vi "Get Absolute XY.vi"(8 "error in (no error)":errorcluster, 10 "Component":T1, 11 "Gantry In":refnum<k24>) -> (0 "error out":errorcluster, 2 "Abs XY":dbl[](array[numeric]), 3 "Gantry Out":refnum<k24>)   [LabVIEW 2021, in "Component Tray.lvclass"]
uses:
  Component Tray.lvclass
  C:/Program Files (x86)/Aerotech/A3200/LabVIEW/2010/Bin/Aerotech.A3200.dll
  Program Files (x86)/Aerotech/A3200/LabVIEW/2010/Bin/Aerotech.A3200.dll
  Find Component.ctl
  Controller/Camera/Machine Vision.ctl
  Component Tray.lvclass/Component Tray.ctl
  Controller/Motion/A3200/A3200.lvclass
  Controller/Camera/Camera.lvclass
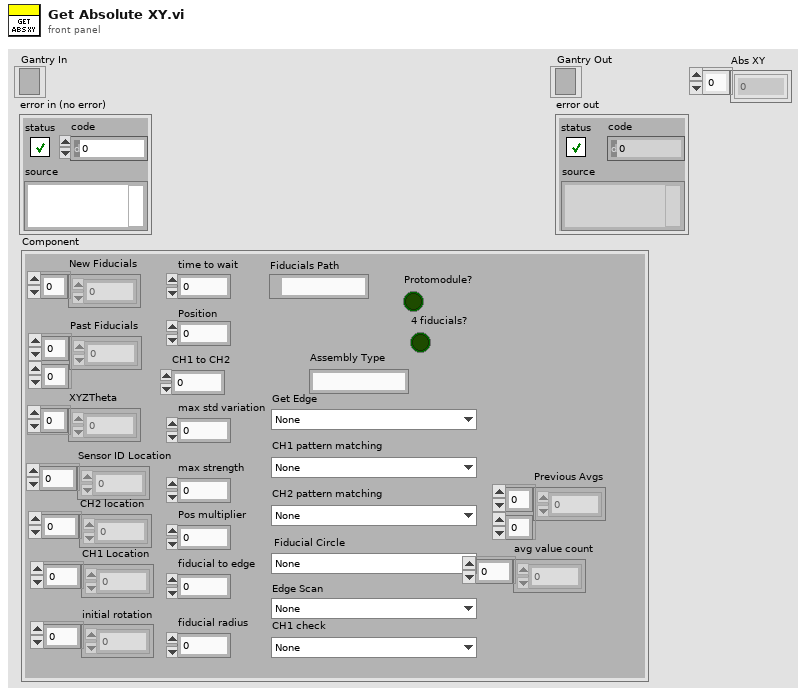
[diagram p1: front panel]
types:
  T1 = typedef "Component Tray.lvclass/Find Component.ctl" = cluster{"New Fiducials":dbl[], "Past Fiducials":dbl[][], "XYZTheta":dbl[], "Fiducials Path":path, "Position":i32, "CH1 Location":dbl[], "Sensor ID Location":dbl[], "initial rotation":dbl[], "CH2 location":dbl[], "max std variation":dbl, "max strength":dbl, "CH2 pattern matching":T2, "Fiducial Circle":T2, "Get Edge":T2, "Pos multiplier":dbl, "time to wait":u32, "fiducial to edge":dbl, "Protomodule?":bool, "Assembly Type":string, "CH1 to CH2":dbl, "Tray Number":string, "fiducial radius":dbl, "4 fiducials?":bool, "CH1 check":T2, "Edge Scan":T2, "CH1 pattern matching":T2, "Sensor Thickness":dbl, "Previous Avgs":dbl[][], "avg value count":dbl[]}
  T2 = typedef "Camera.lvclass/Machine Vision.ctl" = enum16{"None", "Assembly Tray Circle", "Assembly Tray Fiducial", "Partial Hexaboard", "sensor edge init", "HB edge init", "sensor edge pos1", "sensor edge pos2", "HB edge pos1", "HB edge pos2", "Sensor CH1-2", "HB CH1", "HB CH2", "V3 Sensor Circle", "Hexaboard Circle", "sensor CH1 check", "HB CH1 check ", "sensor ID"}
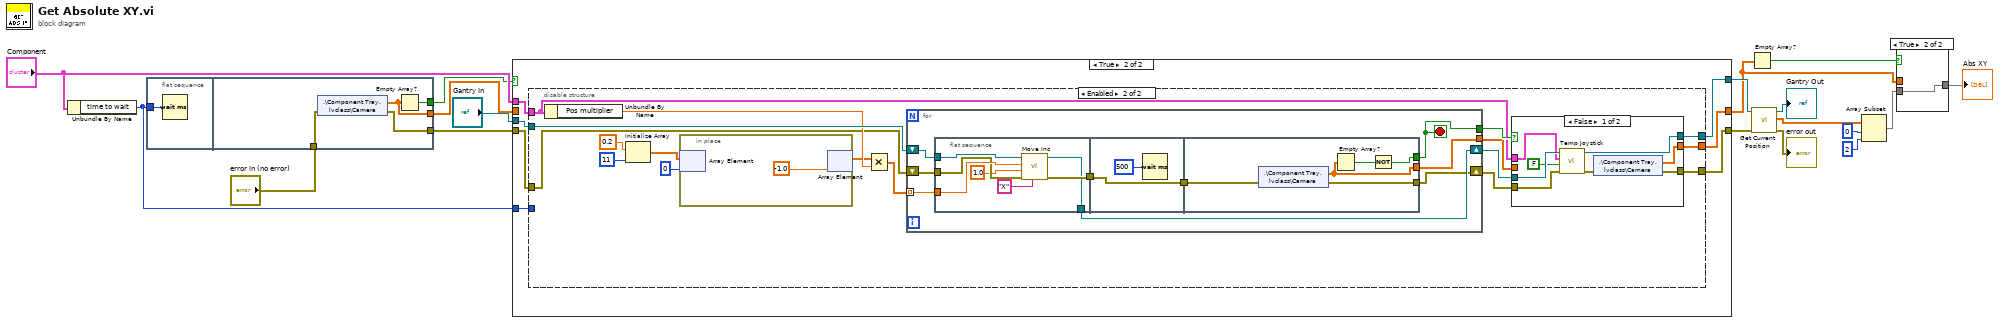
[diagram p0: block diagram]
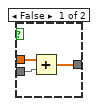
[diagram p2: hidden frame]
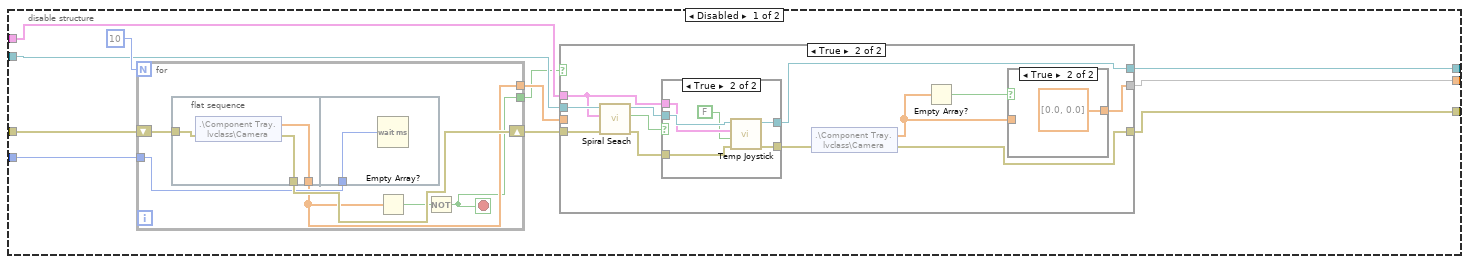
[diagram p4: hidden frame]
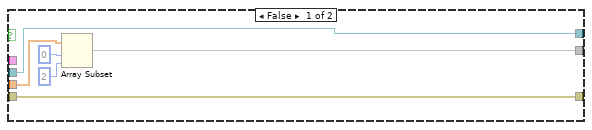
[diagram p5: hidden frame]
diagram:
  n1 = Unbundle By Name("Component") -> ("time to wait"=w11:u32)
  n2 = flat-sequence {
    tunnel: w11 -> [w19]
    tunnel: "error in (no error)" -> [w23]
    tunnel: [w22] -> w9
    tunnel: [w21] -> w8
    tunnel: [w20] -> w7
    frame #0 {
      n3 = Wait (ms)(milliseconds to wait=w19) -> ()  [unwired: 1 out]
    }
    frame #1 {
      n4 = shared-variable ".\\Component Tray.lvclass\\Camera"(error in=w23) -> (w22:dbl[], error out=w21:errorcluster)
      n5 = Empty Array?(array=w22) -> (empty?=w20:bool)
    }
  }
  n6 = case shown="True" w7 {
    tunnel: [w24 w32] -> w2
    tunnel: w8 -> [w26 w33]
    tunnel: [w26 w27] -> w6
    tunnel: w11 -> [_ w31]
    tunnel: "Gantry In" -> [w25 w30]
    tunnel: [w25 w29] -> w12
    tunnel: "Component" -> [_ w28]
    tunnel: w9 -> [w24 _]
    frame False {
    }
    frame True {
      n7 = disable-structure shown="Enabled" {
        disable-tunnel: w33 -> [w43 w96]
        disable-tunnel: [w41 w83] -> w32
        disable-tunnel: w31 -> [w40 _]
        disable-tunnel: w30 -> [w39 w99]
        disable-tunnel: [w38 w93] -> w29
        disable-tunnel: w28 -> [w37 w92]
        disable-tunnel: [w35 w90] -> w27
        frame Disabled {
          n8 = for {
            N: 10 -> [_]
            shift-right: [w49] -> w36
            shift-left: w43 -> [w50]
            tunnel: [w47] -> w42
            tunnel: w40 -> [w48]
            tunnel: [w45] -> w34
            stop <- w45 stop-if-true
            n9 = flat-sequence {
              tunnel: w50 -> [w53]
              tunnel: [w52] -> w49
              tunnel: [w51] -> w47
              tunnel: w48 -> [w54]
              frame #0 {
                n10 = shared-variable ".\\Component Tray.lvclass\\Camera"(error in=w53) -> (w51:dbl[], error out=w52:errorcluster)
              }
              frame #1 {
                n11 = Wait (ms)(milliseconds to wait=w54) -> ()  [unwired: 1 out]
              }
            }
            n12 = Empty Array?(array=w47) -> (empty?=w46:bool)
            n13 = Not(x=w46) -> (.not. x?=w45:bool)
          }
          n14 = case shown="True" w34 {
            tunnel: w42 -> [w58 _]
            tunnel: [w57 w61] -> w41
            tunnel: w39 -> [w56 w72]
            tunnel: [w56 w68] -> w38
            tunnel: w37 -> [_ w66]
            tunnel: w36 -> [w55 w71]
            tunnel: [w55 w64] -> w35
            frame False {
              n15 = Array Subset(array=w58, index=0, length=2) -> (w57:dbl[])
            }
            frame True {
              n16 = call "Spiral Seach.vi"("error in (no error)"=w71, "Component"=w66, "Gantry In"=w72) -> ("error out"=w67:errorcluster, "Error?"=w70:bool, "Gantry Out"=w69:refnum<k24>)  [unwired: 6 in]
              n17 = case shown="True" w70 {
                tunnel: w69 -> [w76 w82]
                tunnel: [w76 w81] -> w68
                tunnel: w67 -> [w75 w80]
                tunnel: [w75 w79] -> w65
                tunnel: w66 -> [_ w78]
                frame False {
                }
                frame True {
                  n18 = call "Temp Joystick.vi"("error in (no error)"=w80, "Fiducial?"=FALSE, "Component"=w78, "Gantry In"=w82) -> ("error out"=w79:errorcluster, "Gantry Out"=w81:refnum<k24>)  [unwired: 5 in, 1 out]
                }
              }
              n19 = shared-variable ".\\Component Tray.lvclass\\Camera"(error in=w65) -> (w62:dbl[], error out=w64:errorcluster)
              n20 = Empty Array?(array=w62) -> (empty?=w63:bool)
              n21 = case shown="True" w63 {
                tunnel: w62 -> [w73 _]
                tunnel: [w73 dbl[] [0.0, 0.0] ("Array of Double")] -> w61
                frame False {
                }
                frame True {
                }
              }
            }
          }
        }
        frame Enabled {
          n22 = Unbundle By Name(w92) -> ("Pos multiplier"=w98:dbl)
          n23 = Initialize Array(0.2 ("element"), 11 ("dimension size")) -> (w87:dbl[])
          n24 = in-place {
            n25 = in-place-array #1(w87, 0) -> ()  [unwired: 1 out]
            n26 = in-place-array #1(-1.0 ("element")) -> (w85:dbl[])  [unwired: 1 out]
          }
          n27 = Multiply(x=w85, y=w98) -> (x*y=w97:dbl[])
          n28 = for {
            tunnel: w97 -> [w117] mode=indexing
            tunnel: [w113] -> w95
            shift-right: [w115] -> w94
            shift-left: w99 -> [w118]
            shift-right: [w114] -> w91
            shift-left: w96 -> [w116]
            tunnel: [w112] -> w84
            stop <- w113 stop-if-true
            n29 = flat-sequence {
              tunnel: w118 -> [w127]
              tunnel: w117 -> [w126]
              tunnel: w116 -> [w125]
              tunnel: [w124] -> w120
              tunnel: [w121] -> w115
              tunnel: w120 -> [w129]
              tunnel: [w129] -> w119
              tunnel: w119 -> [w134]
              tunnel: [w132] -> w113
              tunnel: [w131] -> w114
              tunnel: [w130] -> w112
              frame #0 {
                n30 = call "Move Inc.vi"("Axis"="X", "error in (no error)"=w125, "Speed"=1.0, "Distance"=w126, "Gantry In"=w127) -> ("error out"=w124:errorcluster, "Gantry Out"=w121:refnum<k24>)  [unwired: 5 in]
              }
              frame #1 {
                n31 = Wait (ms)(milliseconds to wait=u32 500) -> ()  [unwired: 1 out]
              }
              frame #2 {
                n32 = shared-variable ".\\Component Tray.lvclass\\Camera"(error in=w134) -> (w130:dbl[], error out=w131:errorcluster)
                n33 = Empty Array?(array=w130) -> (empty?=w133:bool)
                n34 = Not(x=w133) -> (.not. x?=w132:bool)
              }
            }
          }
          n35 = case shown="False" w95 {
            tunnel: w94 -> [w108 w110]
            tunnel: [w107 w110] -> w93
            tunnel: w92 -> [w106 _]
            tunnel: w91 -> [w104 w111]
            tunnel: [w101 w111] -> w90
            tunnel: w84 -> [_ w109]
            tunnel: [w103 w109] -> w83
            frame False {
              n36 = call "Temp Joystick.vi"("error in (no error)"=w104, "Fiducial?"=FALSE, "Component"=w106, "Gantry In"=w108) -> ("error out"=w102:errorcluster, "Gantry Out"=w107:refnum<k24>)  [unwired: 5 in, 1 out]
              n37 = shared-variable ".\\Component Tray.lvclass\\Camera"(error in=w102) -> (w103:dbl[], error out=w101:errorcluster)
            }
            frame True {
            }
          }
        }
      }
    }
  }
  n38 = Empty Array?(array=w2) -> (empty?=w4:bool)
  n39 = call "Get Current Position.vi"("error in (no error)"=w6, "Gantry In"=w12) -> ("error out"=→"error out":errorcluster, "XYZTheta Out"=w18:dbl[], "Gantry Out"=→"Gantry Out":refnum<k24>)  [unwired: 7 in]
  n40 = Array Subset(array=w18, index=0, length=2) -> (w3:dbl[])
  n41 = case shown="True" w4 {
    tunnel: w3 -> [w137 w138]
    tunnel: w2 -> [w136 _]
    tunnel: [w135 w138] -> w1
    frame False {
      n42 = Add(x=w136, y=w137) -> (x+y=w135:dbl[])
    }
    frame True {
    }
  }
  "Abs XY" <- w1
